vi "MouseDown Response.vi"(4 "PlatMods":T1, 6 "Mods":cluster{"Double Click":bool, "Menu Key":bool}, 8 "error in (no error)":errorcluster, 9 "Button":u16, 10 "Coords":T2, 11 "Editor Handler in":refnum<class "Listbox Handler.lvclass">) -> (0 "error out":errorcluster, 3 "Editor Handler out":refnum<class "Listbox Handler.lvclass">)   [LabVIEW 2016, in "Listbox Handler.lvclass"]
uses:
  Listbox Handler.lvclass
  C:/Program Files (x86)/National Instruments/LabVIEW 2016/vi.lib/LIEF/Image Editor Handler/Image Editor Handler.lvclass
  <vilib>/Utility/miscctls.llb/LVPoint32TypeDef.ctl
  <vilib>/LIEF/Image Editor Handler/Image Editor Handler.lvclass/Image Editor Handler.ctl
  Listbox Handler.lvclass/Listbox Handler.ctl
  <vilib>/LIEF/Image Editor Handler/Read Selected.vi
  <vilib>/LIEF/Image Editor Handler/Image Editor Handler.lvclass
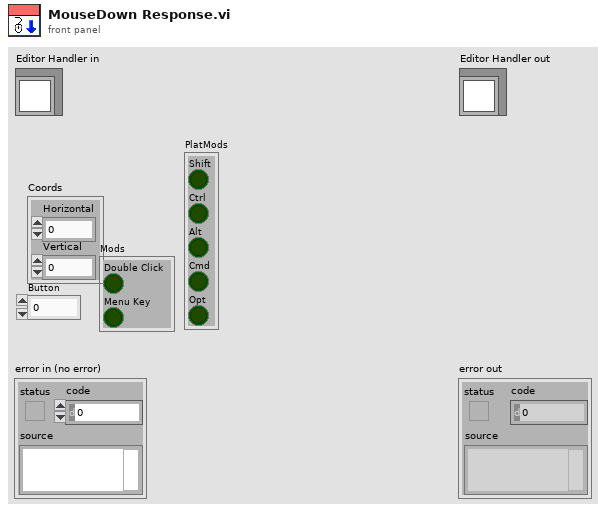
[diagram p1: front panel]
types:
  T1 = cluster{"Shift":bool, "Ctrl":bool, "Alt":bool, "Cmd":bool, "Opt":bool}
  T2 = typedef "LVPoint32TypeDef.ctl" = cluster{"Horizontal":i32, "Vertical":i32}
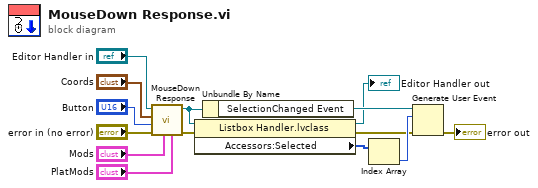
[diagram p0: block diagram]
diagram:
  n1 = call-parent "MouseDown Response.vi"("PlatMods"="PlatMods", "Mods"="Mods", "error in (no error)"="error in (no error)", "Button"="Button", "Coords"="Coords", "Editor Handler in"="Editor Handler in") -> ("error out"=w4:errorcluster, "Editor Handler out"=w7:refnum<class "Listbox Handler.lvclass">)  [unwired: 4 in]
  n2 = property class="Listbox Handler.lvclass"(reference=w7, error in=w4) -> (reference out=→"Editor Handler out":refnum<class "Listbox Handler.lvclass">, error out=w3:errorcluster, "Accessors:Selected"=w8:i16[])
  n3 = Unbundle By Name(w7) -> ("SelectionChanged Event"=w6:refnum<user-event>)
  n4 = Index Array(array=w8) -> (element=w5:i16)  [unwired: 1 in]
  n5 = Generate User Event(user event=w6, event data cluster=w5, error in=w3) -> (error out=→"error out":errorcluster)  [unwired: 1 in, 1 out]
